vi "Encoder Throwout.vi"(11 "Input":dbl) -> (3 "Output":dbl)   [LabVIEW 2016]
panel:
  out "Under max?":bool
  in  "Range":dbl
  out "Passed?":bool
  out "Value Rejection History":i16(graph)=1
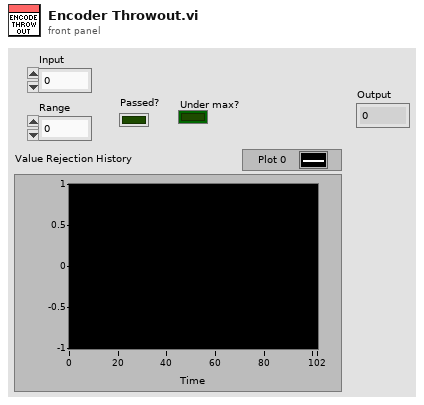
[diagram p1: front panel]
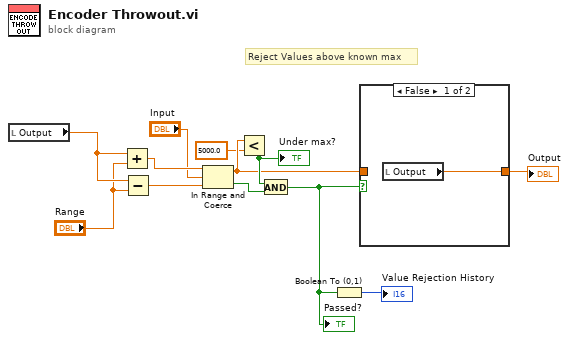
[diagram p0: block diagram]
diagram:
  # "Reject Values above known max"
  n1 = local read "Output"() -> (w3:dbl)
  n2 = Add(x=w3, y="Range") -> (x+y=w12:dbl)
  n3 = Subtract(x=w3, y="Range") -> (x-y=w11:dbl)
  n4 = In Range and Coerce(upper limit=w12, x="Input", lower limit=w11) -> (coerced(x)=w4:dbl, In Range?=w9:bool)
  n5 = Less?(x=w4, y=5000.0) -> (x < y?=w5:bool)
  "Under max?" <- w5
  n6 = And(x=w5, y=w9) -> (x .and. y?=w6:bool)
  "Passed?" <- w6
  n7 = Boolean To (0,1)(Boolean=w6) -> (0, 1=→"Value Rejection History":i16)
  n8 = case shown="False" w6 {
    tunnel: [w13 w14] -> w7
    tunnel: w4 -> [_ w14]
    frame False {
      n9 = local read "Output"() -> (w13:dbl)
    }
    frame True {
    }
  }
  "Output" <- w7
